vi "Hello World.vi"() -> ()   [LabVIEW 2016]
panel:
  in  "stop":bool
  out "Text window":string
  out "Led":bool
  in  "Button":bool
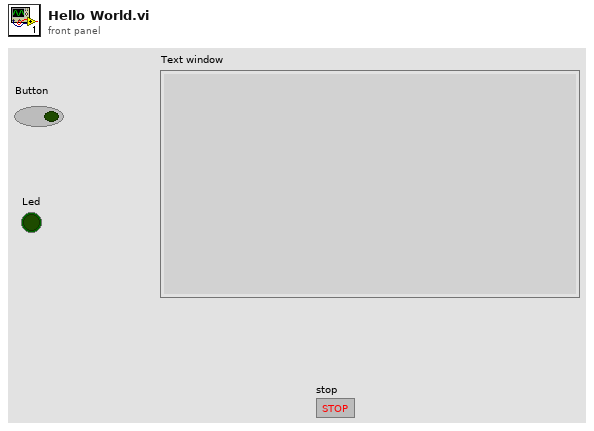
[diagram p1: front panel]
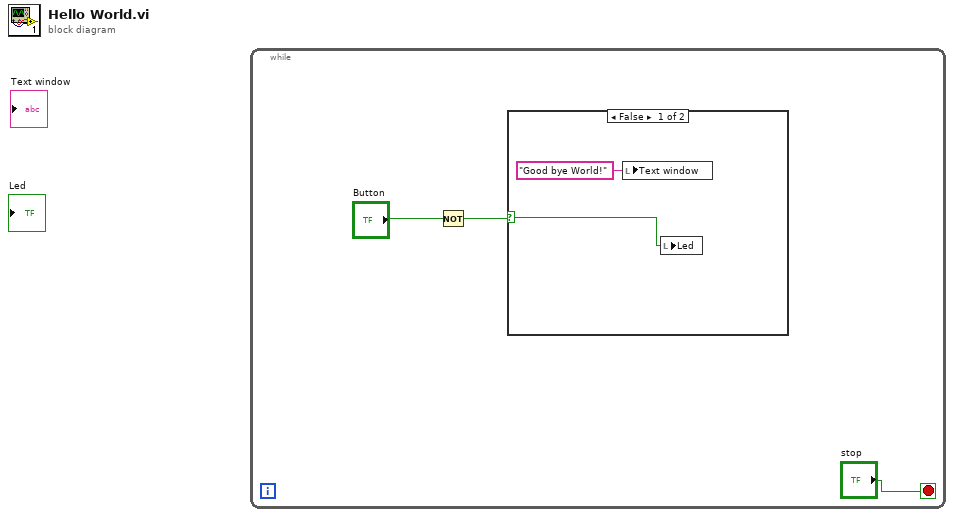
[diagram p0: block diagram]
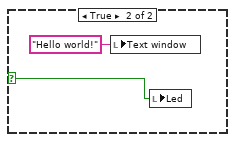
[diagram p2: hidden frame]
diagram:
  n1 = while {
    stop <- "stop" stop-if-true
    n2 = Not(x="Button") -> (.not. x?=w2:bool)
    n3 = case shown="False" w2 {
      selector: w2 -> [w4 w6]
      frame False {
        n4 = local write "Text window"("Good bye World!" ("Text window")) -> ()
        n5 = local write "Led"(w4) -> ()
      }
      frame True {
        n6 = local write "Text window"("Hello world!" ("Text window")) -> ()
        n7 = local write "Led"(w6) -> ()
      }
    }
  }
